vi "String To Hex（两位 ）.vi"(11 "String":string) -> (2 "Out":string, 3 "Hex":string)   [LabVIEW 2014]
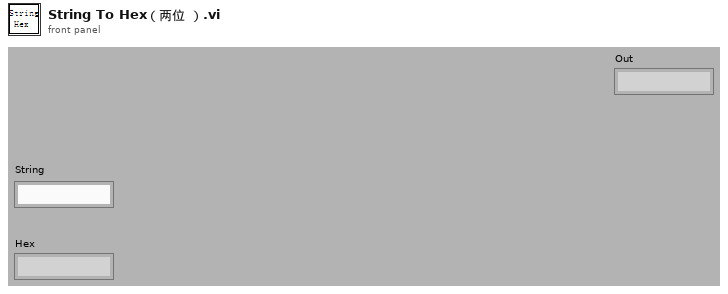
[diagram p1: front panel]
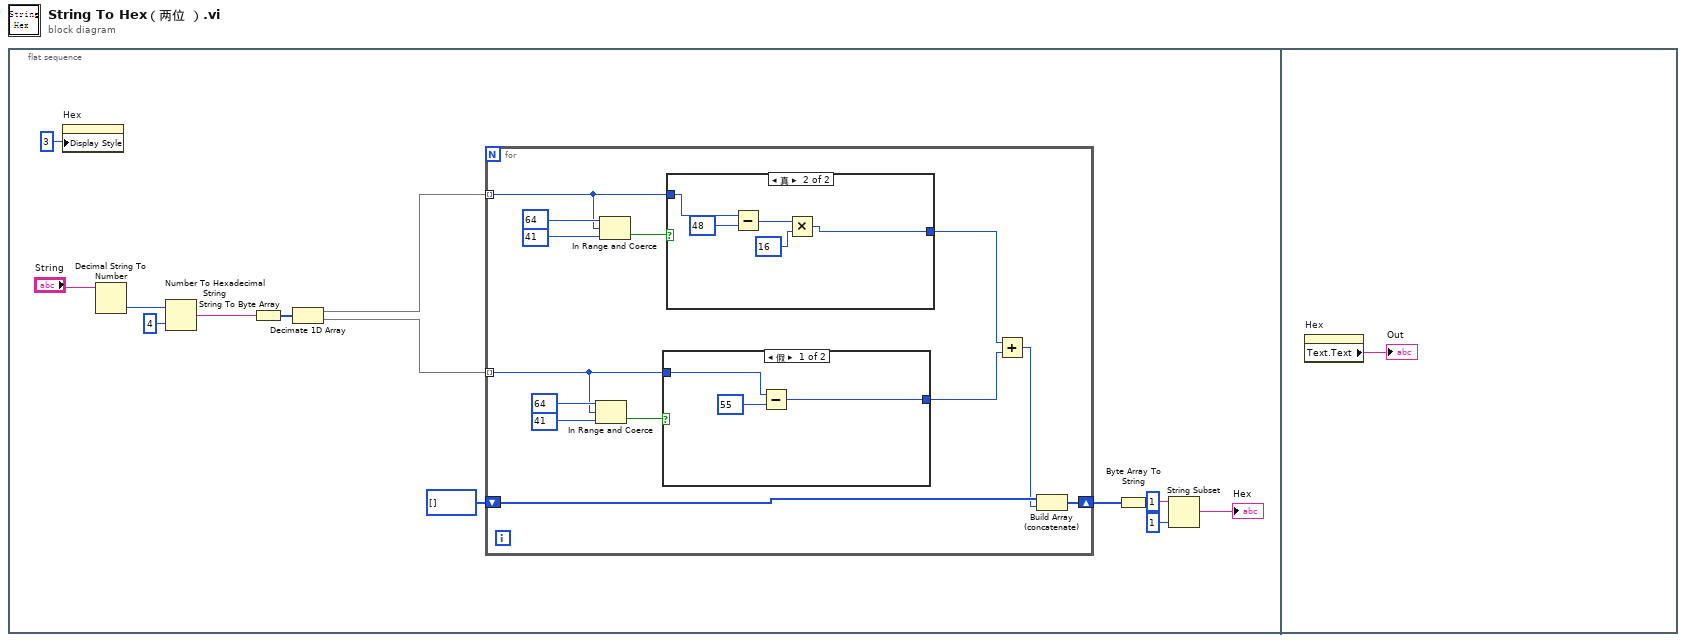
[diagram p0: block diagram]
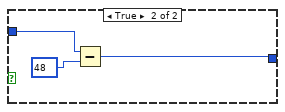
[diagram p2: hidden frame]
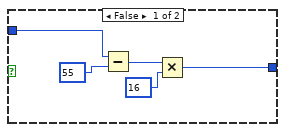
[diagram p3: hidden frame]
diagram:
  n1 = flat-sequence {
    frame #0 {
      n2 = property on="Hex" class="Str"("Display Style"=u32 3 ("显示样式")) -> ()  [unwired: 2 in, 2 out]
      n3 = Decimal String To Number(string="String") -> (number=w13:i32)  [unwired: 2 in, 1 out]
      n4 = Number To Hexadecimal String(1:i16 4 ("宽度(-)"), 2:w13) -> (0:w7:string)
      n5 = String To Byte Array(string=w7) -> (unsigned byte array=w10:u8[])
      n6 = Decimate 1D Array(w10) -> (w9:u8[], w8:u8[])
      n7 = for {
        shift-right: [w17] -> w5
        shift-left: u8[] [] -> [w19]
        tunnel: w9 -> [w16] mode=indexing
        tunnel: w8 -> [w15] mode=indexing
        n8 = In Range and Coerce(upper limit=u8 64 ("上限"), x=w15, lower limit=u8 41 ("下限")) -> (In Range?=w22:bool)  [unwired: 1 out]
        n9 = In Range and Coerce(upper limit=u8 64 ("上限"), x=w16, lower limit=u8 41 ("下限")) -> (In Range?=w25:bool)  [unwired: 1 out]
        n10 = case shown="假" w22 {
          tunnel: w15 -> [w28 w32]
          tunnel: [w29 w31] -> w20
          frame False {
            n11 = Subtract(x=w28, y=u8 55 ("上限")) -> (x-y=w29:u8)
          }
          frame True {
            n12 = Subtract(x=w32, y=u8 48 ("上限")) -> (x-y=w31:u8)
          }
        }
        n13 = case shown="真" w25 {
          tunnel: w16 -> [w35 w39]
          tunnel: [w34 w40] -> w21
          frame False {
            n14 = Subtract(x=w35, y=u8 55 ("上限")) -> (x-y=w37:u8)
            n15 = Multiply(x=w37, y=u8 16 ("上限")) -> (x*y=w34:u8)
          }
          frame True {
            n16 = Subtract(x=w39, y=u8 48 ("上限")) -> (x-y=w42:u8)
            n17 = Multiply(x=w42, y=u8 16 ("上限")) -> (x*y=w40:u8)
          }
        }
        n18 = Add(x=w21, y=w20) -> (x+y=w18:u8)
        n19 = Build Array (concatenate)(w19, w18) -> (w17:u8[])
      }
      n20 = Byte Array To String(unsigned byte array=w5) -> (string=w4:string)
      n21 = String Subset(string=w4, offset (0)=1 ("偏移量(0)"), length (rest)=1 ("长度（剩余）")) -> (substring=→"Hex":string)
    }
    frame #1 {
      n22 = property on="Hex" class="Str"() -> ("Text.Text"=→"Out":string)  [unwired: 2 in, 2 out]
    }
  }
